vi "FTW-TransferClient-GetHeaders.vi"(1 "Transfer Client":refnum<class "FTW-TransferClient.lvclass">) -> (0 "Headers":T1[](array[typedef]))   [LabVIEW 2012, in "FTW-TransferClient.lvclass"]
uses:
  FTW-TransferClient.lvclass
  Core/Collection/FTW-Collection-KeyValuePair.ctl
  FTW-TransferClient.lvclass/FTW-TransferClient.ctl
panel:
  # "Inputs"
  # "Outputs"
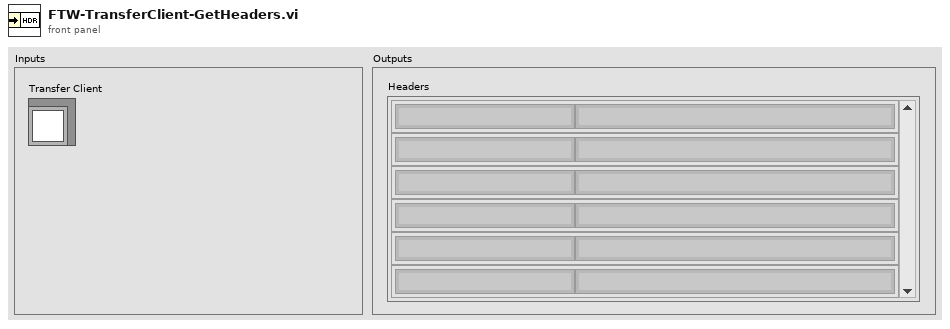
[diagram p1: front panel]
types:
  T1 = typedef "FTW-Collection-KeyValuePair.ctl" = cluster{"Key":string, "Value":string}
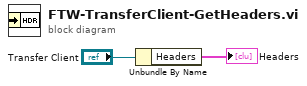
[diagram p0: block diagram]
diagram:
  n1 = Unbundle By Name("Transfer Client") -> ("Headers"=→"Headers":T1[])
